vi "New JSON Null.vi"(8 "error in (no error)":errorcluster) -> (0 "error out":errorcluster, 3 "JSON String out":refnum<class "JSON Null.lvclass">)   [LabVIEW 2017, in "LVJSON.lvlib" / "JSON Null.lvclass"]
uses:
  JSON Null.lvclass
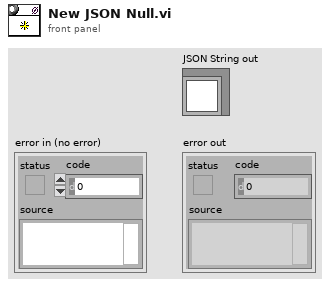
[diagram p1: front panel]
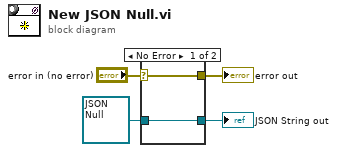
[diagram p0: block diagram]
diagram:
  n1 = case shown="No Error" "error in (no error)" {
    selector: "error in (no error)" -> [w5 w8]
    tunnel: [w5 w8] -> w3
    tunnel: [w6 w7] -> w1
    tunnel: refnum<class "JSON Null.lvclass"> refnum ("JSON String in") -> [w6 w7]
    frame No Error {
    }
    frame Error {
    }
  }
  "error out" <- w3
  "JSON String out" <- w1
